vi "initialize PQ and visited list.vi"(11 "start state":refnum<data-value>) -> (2 "Astar Open List out":refnum<class "NI_Robotics_Priority Queue.lvclass">, 3 "visited list":variant)   [LabVIEW 2017, in "NI_Robotics_Navigation .lvlib"]
uses:
  <vilib>/robotics/Navigation/NI_Robotics_Navigation .lvlib
  <vilib>/robotics/Navigation/shared/Priority Queue/NI_Robotics_Priority Queue.lvclass
  <vilib>/robotics/Navigation/shared/MapNode/AbstractMapNode/NI_Robotics_AbstractMapNode.lvclass
  <vilib>/robotics/Navigation/shared/Priority Queue/Open List Element.ctl
  <vilib>/robotics/Navigation/Astar/Visited List Element.ctl
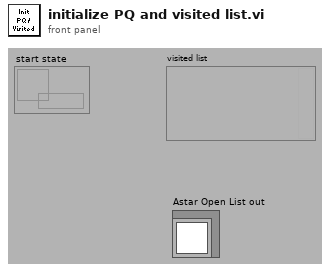
[diagram p1: front panel]
types:
  T1 = typedef "NI_Robotics_Navigation .lvlib/Visited List Element.ctl" = cluster{"Best cost to state":dbl, "Back pointer":refnum<data-value>}
  T2 = typedef "NI_Robotics_Priority Queue.lvclass/Open List Element.ctl" = cluster{"f":dbl, "g":dbl, "node Ref":refnum<data-value>}
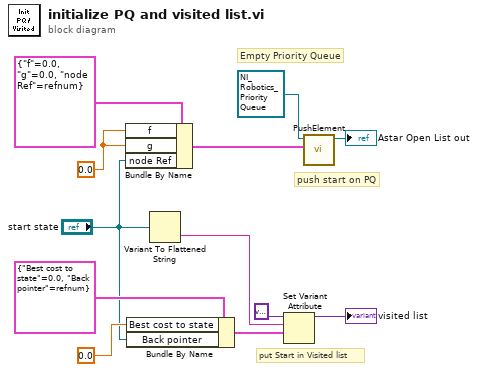
[diagram p0: block diagram]
diagram:
  w7 = 0.0 ("f(State)")
  # "push start on PQ"
  # "put Start in Visited list"
  # "Empty Priority Queue"
  n1 = Bundle By Name(cluster=T2 {"f"=0.0, "g"=0.0, "node Ref"=refnum} ("Open List Element"), "f"=w7, "g"=w7, "node Ref"="start state") -> (w3:T2)
  n2 = Bundle By Name(cluster=T1 {"Best cost to state"=0.0, "Back pointer"=refnum} ("Visited List Element"), "Best cost to state"=0.0, "Back pointer"="start state") -> (w9:T1)
  n3 = Variant To Flattened String(Variant="start state") -> (data string=w6:string)  [unwired: 1 out]
  n4 = Set Variant Attribute(Variant=variant ("variant"), name=w6, value=w9) -> (Variant out=→"visited list":variant)  [unwired: 1 in, 2 out]
  n5 = call <vilib>:"PushElement.vi"("open list element"=w3, "Astar Open List in"=refnum<class "NI_Robotics_Priority Queue.lvclass"> refnum ("NI_Robotics_Navigation .lvlib:Priority Queue.lvclass")) -> ("Astar Open List out"=→"Astar Open List out":refnum<class "NI_Robotics_Priority Queue.lvclass">)  [unwired: 8 in, 1 out]
